vi "swmm_get_mass_bal_error.vi"(6 "error in (no error)":errorcluster) -> (0 "error out":errorcluster, 1 "qual_error":sgl, 2 "flow_error":sgl, 3 "runoff_error":sgl)   [LabVIEW 2014]
uses:
  swmm5.dll
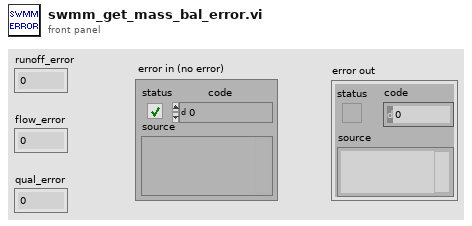
[diagram p1: front panel]
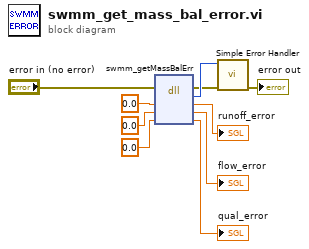
[diagram p0: block diagram]
diagram:
  n1 = dll-call lib="PTH2zabs CUsers\nandres riañoDropboxProyecto AguasSoftwareMatSWMMMatSWMM 5.1.009LabVIEW modulex64\tswmm5.dll" fn="swmm_getMassBalErr"(error in="error in (no error)", "runoff_error"=sgl 0.0, "flow_error"=sgl 0.0 ("runoff_error"), "qual_error"=sgl 0.0 ("runoff_error")) -> (error out=w3:errorcluster, "return type"=w10:i32, "runoff_error"=→"runoff_error":sgl, "flow_error"=→"flow_error":sgl, "qual_error"=→"qual_error":sgl)  [unwired: 2 in, 1 out]
  n2 = call <vilib>:"Simple Error Handler.vi"("error code (no error:0)"=w10, "error in (no error)"=w3) -> ("error out"=→"error out":errorcluster)  [unwired: 3 in, 4 out]
